vi "TwTpsGetModuleLimits.vi"(0 "moduleCode":i32, 1 "error in (no error)":errorcluster) -> (2 "maxLimit":dbl, 3 "minLimit":dbl, 4 "error out":errorcluster)   [LabVIEW 2009]
uses:
  TofDaqDll.dll
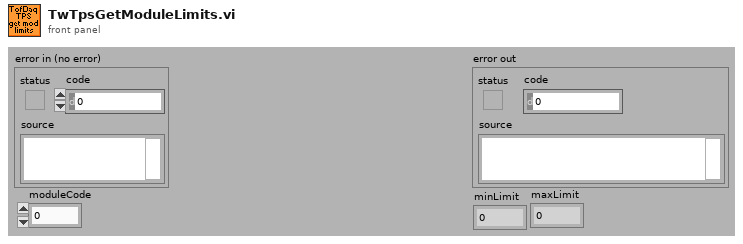
[diagram p1: front panel]
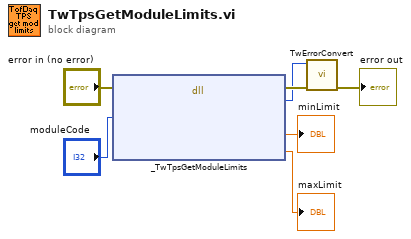
[diagram p0: block diagram]
diagram:
  n1 = dll-call lib="C:/src/TofDaq/APIandWrappers/LabView/TofDaqDll/TofDaqDll.dll" fn="_TwTpsGetModuleLimits"(error in="error in (no error)", "moduleCode"="moduleCode") -> (error out=w6:errorcluster, "TwRetVal"=w4:i32, "minLimit"=→"minLimit":dbl, "maxLimit"=→"maxLimit":dbl)  [unwired: 2 in, 4 out]
  n2 = call "TwErrorConvert.vi"("error in (no error)"=w6, "error code"=w4) -> ("error out"=→"error out":errorcluster)  [unwired: 9 out]
